vi "EncoderPosition.vi"() -> ()   [LabVIEW 2010]
uses:
  <vilib>/NXT/Subs/MotorXNode.DC Motor Type.ctl
  <vilib>/NXT/Subs/LVHSConnector.ctl
  <vilib>/NXT/NXTIO Xnodes/NXTIOXNode/NXTIO.xnode
  <vilib>/NXT/Subs/MotorXNode.2DCMotor.ctl
  <vilib>/NXT/NXTIO Xnodes/NXTIONodeSubVIs/TETRIX IO Reset Encoders.vi
  <vilib>/NXT/NXTIO Xnodes/NXTIONodeSubVIs/TETRIX IO Move DC Motors.vi
  <vilib>/NXT/NXTIO Xnodes/NXTIONodeSubVIs/TETRIX IO Motor Status.vi
  <vilib>/NXT/NXTIO Xnodes/NXTIONodeSubVIs/TETRIX IO Stop DC Motors.vi
panel:
  in  "Encoder Motor":T2
  in  "Both Lift":T2
  in  "Power":i8
  in  "Position":i32
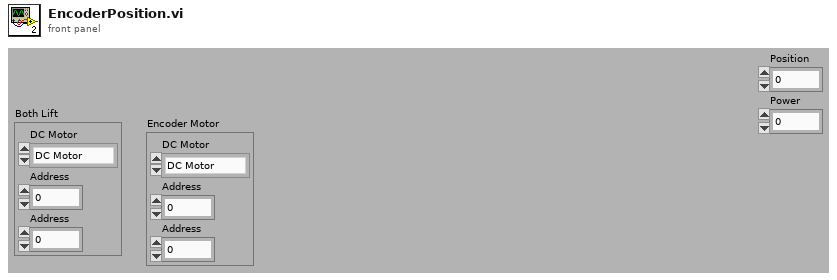
[diagram p1: front panel]
types:
  T1 = typedef "MotorXNode.DC Motor Type.ctl" = enum16{"DC Motor"}
  T2 = cluster{"DC Motor":T1, "Address":i16, "Address":i16}
  T3 = typedef "LVHSConnector.ctl" = cluster{"Hardware":string, "Flattened String":string}
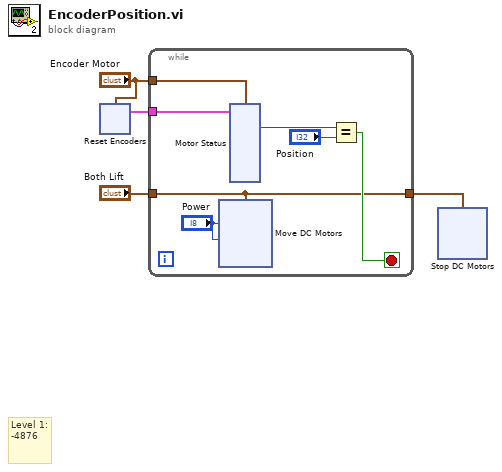
[diagram p0: block diagram]
diagram:
  # "Level 1:\n-4876"
  n1 = xnode "Reset Encoders"("Motors"="Encoder Motor") -> ("NXT"=w4:T3)  [unwired: 1 in]
  n2 = while {
    tunnel: "Encoder Motor" -> [w11]
    tunnel: w4 -> [w8]
    tunnel: "Both Lift" -> [w5]
    tunnel: [w5] -> w1
    stop <- w7 stop-if-true
    n3 = xnode "Move DC Motors"("Power/Speed 2"="Power", "Power/Speed 1"="Power", "Motors"=w5) -> ()  [unwired: 1 in, 1 out]
    n4 = xnode "Motor Status"("Motors"=w11, "NXT"=w8) -> ("Position 1"=w10:i32)  [unwired: 4 out]
    n5 = Equal?(x=w10, y="Position") -> (x = y?=w7:bool)
  }
  n6 = xnode "Stop DC Motors"("Motors"=w1) -> ()  [unwired: 1 in, 1 out]
